vi "Write Elapsed Time Ref.vi"(6 "Elapsed Time Ref":refnum<vi>, 11 "Active Station Time Remaining View Definition in":refnum<class "Active Option Elapsed Time View Definition.lvclass">) -> (3 "Active Station Time Remaining View Definition out":refnum<class "Active Option Elapsed Time View Definition.lvclass">)   [LabVIEW 2019, in "Active Option Elapsed Time View Definition.lvclass"]
uses:
  <vilib>/gpm_packages/@cs/Car-wash/Source/Active Station Time Remaining View Definition/Active Station Time Remaining View Definition/Active Option Elapsed Time View Definition.lvclass
  <vilib>/gpm_packages/@cs/Car-wash/Source/Active Station Time Remaining View Definition/Active Station Time Remaining View Definition/Active Option Elapsed Time View Definition.lvclass/Active Option Elapsed Time View Definition.ctl
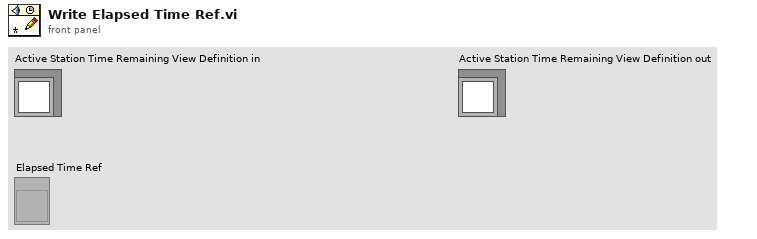
[diagram p1: front panel]
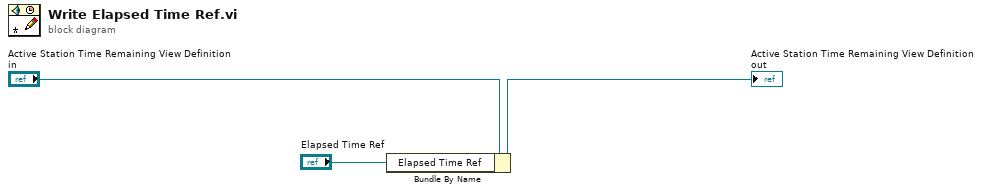
[diagram p0: block diagram]
diagram:
  n1 = Bundle By Name(cluster="Active Station Time Remaining View Definition in", "Elapsed Time Ref"="Elapsed Time Ref") -> (→"Active Station Time Remaining View Definition out":refnum<class "Active Option Elapsed Time View Definition.lvclass">)
